vi "Send Clear History.vi"(0 "Message Enqueuer":refnum<class "Message Enqueuer.lvclass">, 5 "error in (no error)":errorcluster, 6 "Actor Name":string, 7 "Callback Queue":refnum<queue>, 8 "Message Priority (Normal)":T1=enum."Normal", 9 "timeout in ms (-1)":i32) -> (13 "TimeOut":bool, 14 "Message Enqueuer out":refnum<class "Message Enqueuer.lvclass">, 19 "error out":errorcluster)   [LabVIEW 2019, in "BNT_XtGraph.lvlib" / "Clear History Msg.lvclass"]
doc: "Sends the <B>BNT_XtGraph.lvlib:Clear History Msg.lvclass</B> message.\n\n<B>BNT_XtGraph.lvlib:BNT_XtGraph.lvclass:Clear History.vi</B> Description:\n\nClear history data."
uses:
  Clear History Msg.lvclass
  <vilib>/ActorFramework/Message Enqueuer/Message Enqueuer.lvclass
  <vilib>/ActorFramework/Message Enqueuer/Message Priority.ctl
  C:/User/Brand/LVP/LaserSpec/RADRIS/Packages/CSPP_Core/Messages/CSPP_AsyncCallbackMsg/CSPP_AsyncCallback Msg.lvclass
  C:/Program Files (x86)/National Instruments/LabVIEW 2019/vi.lib/ActorFramework/Message/Message.lvclass
  CSPP_Core/Messages/CSPP_AsyncCallbackMsg/CSPP_AsyncCallback Msg.lvclass/CSPP_AsyncCallback Msg.ctl
  <vilib>/ActorFramework/Message Enqueuer/Message Enqueuer.lvclass/Message Enqueuer.ctl
  <vilib>/ActorFramework/Message Priority Queue/Priority Enqueue.vi
  CSPP_Core/Messages/CSPP_AsyncCallbackMsg/CSPP_AsyncCallback Msg.lvclass
  CSPP_Core/Libraries/Utilities/CSPP_Utilities.lvlib
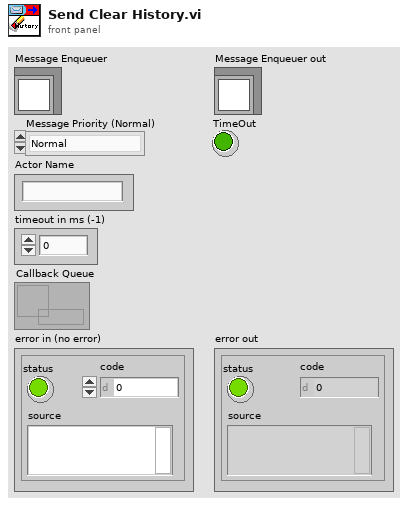
[diagram p1: front panel]
types:
  T1 = typedef "Actor Framework.lvlib/Message Enqueuer.lvclass/Message Priority.ctl" = enum16{"Low", "Normal", "High"}
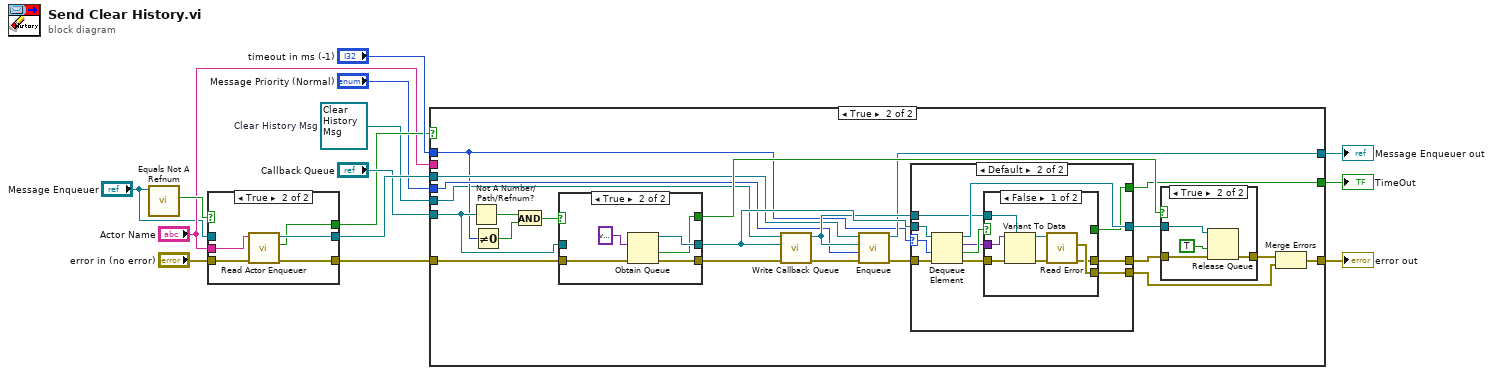
[diagram p0: block diagram]
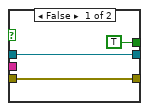
[diagram p2: hidden frame]
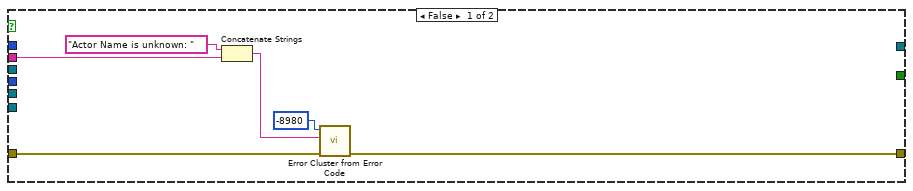
[diagram p3: hidden frame]
diagram:
  w1 = refnum<class "Clear History Msg.lvclass"> refnum  # Clear History Msg
  n1 = call <vilib>:"Equals Not A Refnum.vi"("Message Enqueuer"="Message Enqueuer") -> ("Not a refnum?"=w14:bool)  [unwired: 10 in]
  n2 = case shown="True" w14 {
    tunnel: "error in (no error)" -> [w16 w22]
    tunnel: [w16 w21] -> w13
    tunnel: "Actor Name" -> [_ w18]
    tunnel: [w17 w20] -> w12
    tunnel: "Message Enqueuer" -> [w17 _]
    tunnel: [TRUE ("Success") w19] -> w8
    frame False {
    }
    frame True {
      n3 = call "Read Actor Enqueuer.vi"("Error In"=w22, "Actor Name"=w18) -> ("Error Out"=w21:errorcluster, "Success"=w19:bool, "Enqueuer"=w20:refnum<class "Message Enqueuer.lvclass">)  [unwired: 6 in, 1 out]
    }
  }
  n4 = case shown="True" w8 {
    tunnel: w13 -> [w28 w40]
    tunnel: w12 -> [_ w39]
    tunnel: "Message Priority (Normal)" -> [_ w38]
    tunnel: "Callback Queue" -> [_ w31]
    tunnel: [_ w37] -> w4
    tunnel: [w27 w36] -> w5
    tunnel: [_ w35] -> w10
    tunnel: "timeout in ms (-1)" -> [_ w30]
    tunnel: "Actor Name" -> [w23 _]
    tunnel: w1 -> [_ w29]
    frame False {
      n5 = Concatenate Strings("Actor Name is unknown: " ("Error Message (\"\")"), w23) -> (w24:string)
      n6 = call "Error Cluster from Error Code.vi"("Error In"=w28, "Error Message (\"\")"=w24, "Error Code (0)"=-8980) -> ("Error Out"=w27:errorcluster)  [unwired: 8 in]
    }
    frame True {
      n7 = Not A Number/Path/Refnum?(number/path/refnum=w31) -> (NaN/Path/Refnum?=w34:bool)
      n8 = Not Equal To 0?(x=w30) -> (x != 0?=w33:bool)
      n9 = And(x=w34, y=w33) -> (x .and. y?=w32:bool)
      n10 = case shown="True" w32 {
        tunnel: w31 -> [w74 _]
        tunnel: [w74 w79] -> w48
        tunnel: [w73 w77] -> w49
        tunnel: w40 -> [w73 w76]
        tunnel: [_ w75] -> w46
        frame False {
        }
        frame True {
          n11 = Obtain Queue(element data type=variant, error in (no error)=w76) -> (queue out=w79:refnum<queue>, created new?=w75:bool, error out=w77:errorcluster)  [unwired: 3 in]
        }
      }
      n12 = call "Write Callback Queue.vi"("error in (no error)"=w49, "Callback Queue"=w48, "CSPP_AsyncCallback Msg in"=w29) -> ("error out"=w50:errorcluster, "CSPP_AsyncCallback Msg out"=w42:refnum<class "Clear History Msg.lvclass">)  [unwired: 7 in]
      n13 = call <vilib>:"Enqueue.vi"("error in (no error)"=w50, "Message Priority (Normal)"=w38, "Message"=w42, "Message Enqueuer in"=w39) -> ("error out"=w47:errorcluster, "Message Enqueuer out"=w37:refnum<class "Message Enqueuer.lvclass">)  [unwired: 6 in]
      n14 = case shown="Default" w30 {
        selector: w30 -> [_ w60]
        tunnel: w48 -> [w52 w61]
        tunnel: [w52 w63] -> w45
        tunnel: [w51 w53] -> w44
        tunnel: w47 -> [w51 w62]
        tunnel: w42 -> [_ w57]
        tunnel: [_ w55] -> w35
        tunnel: [_ w54] -> w41
        frame 0 {
        }
        frame Default {
          n15 = Dequeue Element(queue=w61, timeout in ms (-1)=w60, error in (no error)=w62) -> (queue out=w63:refnum<queue>, element=w58:variant, timed out?=w59:bool, error out=w56:errorcluster)
          n16 = case "Dequeue Case" shown="False" w59 {
            selector: w59 -> [_ w72]
            tunnel: w58 -> [w70 _]
            tunnel: w57 -> [w69 _]
            tunnel: w56 -> [w68 w71]
            tunnel: [_ w72] -> w55
            tunnel: [w65 _] -> w54
            tunnel: [w64 w71] -> w53
            frame False {
              n17 = Variant To Data(error in=w68, type=w69, Variant=w70) -> (data=w67:refnum<class "Clear History Msg.lvclass">, error out=w66:errorcluster)
              n18 = call "Read Error.vi"("error in (no error)"=w66, "CSPP_AsyncCallback Msg in"=w67) -> ("error out"=w64:errorcluster, "Error"=w65:errorcluster)  [unwired: 7 in, 1 out]
            }
            frame True {
            }
          }
        }
      }
      n19 = case shown="True" w46 {
        tunnel: w45 -> [_ w84]
        tunnel: w44 -> [w80 w83]
        tunnel: [w80 w81] -> w43
        frame False {
        }
        frame True {
          n20 = Release Queue(queue=w84, force destroy? (F)=TRUE, error in (no error)=w83) -> (error out=w81:errorcluster)  [unwired: 2 out]
        }
      }
      n21 = Merge Errors(w43, w41) -> (w36:errorcluster)
    }
  }
  "error out" <- w5
  "Message Enqueuer out" <- w4
  "TimeOut" <- w10
